vi "CHART_GRAPH_EXAMPLE.vi"() -> ()   [LabVIEW 2018]
panel:
  out "Waveform Graph":i32[](graph)
  out "Numeric 2":i32
  out "Array":i32[](array[numeric])
  in  "Numeric":i32
  out "Waveform Chart":i32(graph)
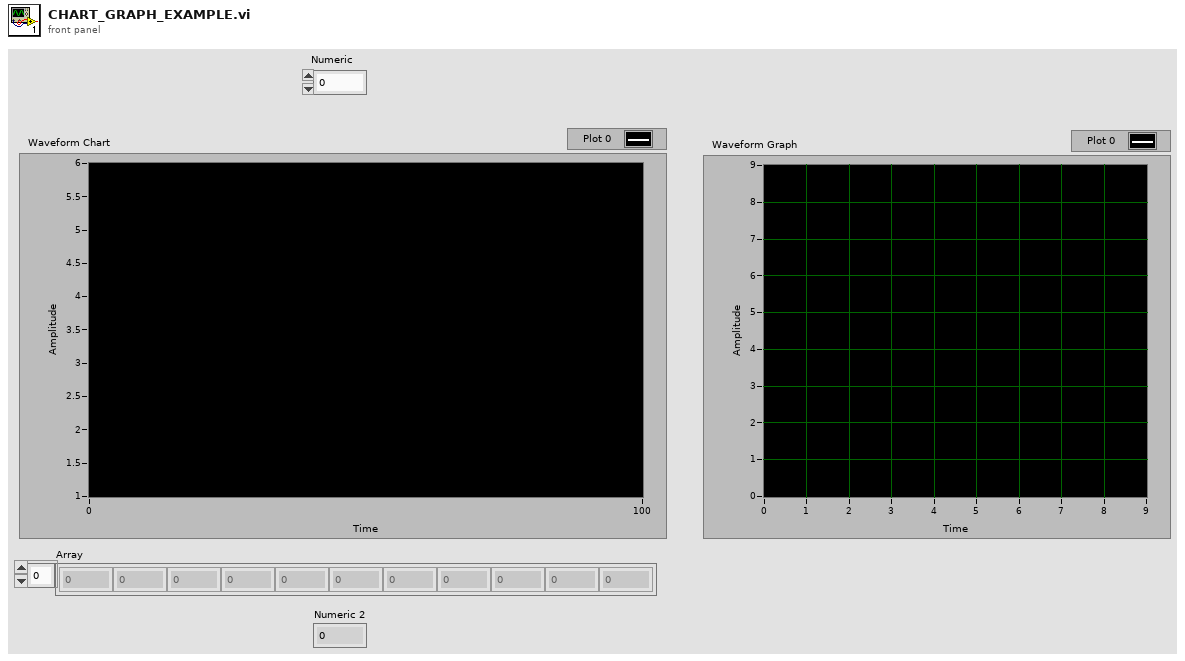
[diagram p1: front panel]
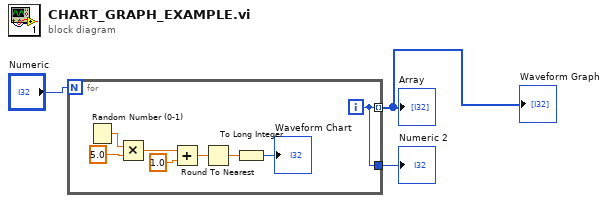
[diagram p0: block diagram]
diagram:
  n1 = for {
    N: "Numeric" -> [_]
    tunnel: [w4] -> w1 mode=indexing
    tunnel: [w4] -> w2
    i -> [w4]
    n2 = Random Number (0-1)() -> (number: 0 to 1=w10:dbl)
    n3 = Multiply(x=w10, y=5.0) -> (x*y=w9:dbl)
    n4 = Add(x=w9, y=1.0) -> (x+y=w7:dbl)
    n5 = Round To Nearest(number=w7) -> (nearest integer value=w6:dbl)
    n6 = To Long Integer(number=w6) -> (32bit integer=→"Waveform Chart":i32)
  }
  "Array" <- w1
  "Numeric 2" <- w2
  "Waveform Graph" <- w1
